vi "tsdb_get_flexray_ecu_properties_by_address_verbose.vi"(8 "error in (no error)":errorcluster caption="错误输入（无错误）", 10 "AAddr":string, 11 "path in":path) -> (0 "error out":errorcluster caption="错误输出", 1 "flexray_ecu_properties_by_address":T1, 2 "function return":i32, 3 "path out":path)   [LabVIEW 2014]
doc: "Function introduction: Obtain Flexray ECU attribute information through address\nCall location\nInput parameter Adder: Address\nADBIndex：\n Database index\nAECUIndex：\n Number of returned signals\nATxFrameCount：\n Returned TX frame rate\nARxFrameCount：\n The number of Rx frames returned\nAName：\n Database Name\nAComment：\n notes\nReturn value 0: Successful execution\nOther values: Failed"
uses:
  Typedef/FlexRay/flexray_ecu_properties_by_address.ctl
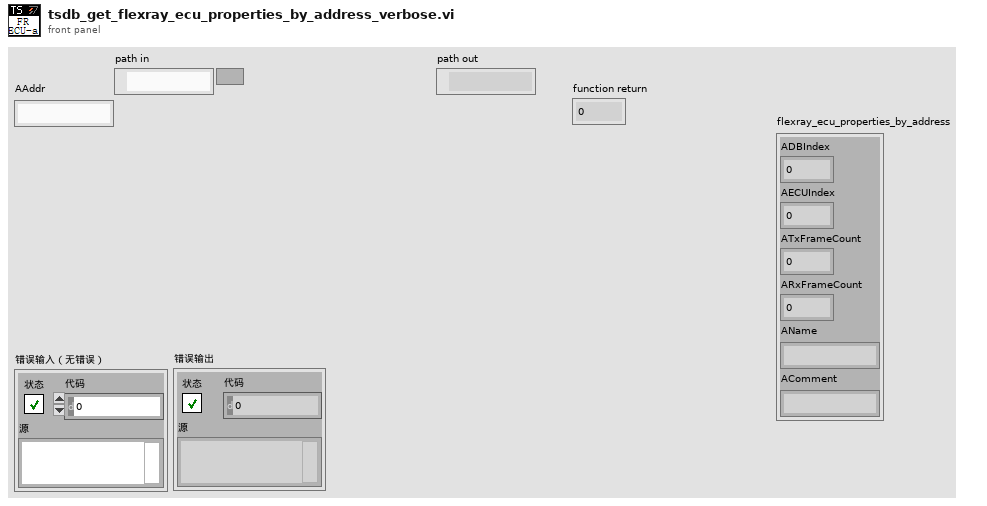
[diagram p1: front panel]
types:
  T1 = typedef "flexray_ecu_properties_by_address.ctl" = cluster{"ADBIndex":i32, "AECUIndex":i32, "ATxFrameCount":i32, "ARxFrameCount":i32, "AName":string, "AComment":string}
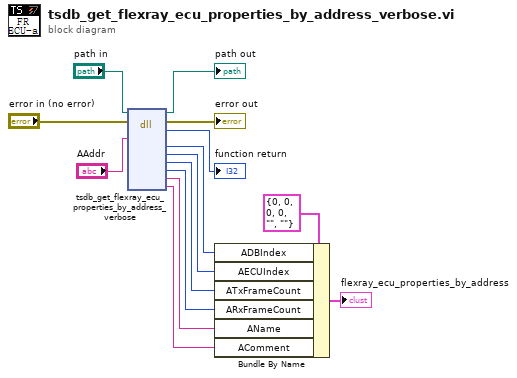
[diagram p0: block diagram]
diagram:
  n1 = dll-call lib="D:/Work/LabVIEW Code/TSMaster Labview SDK/LabVIEW/LabVIEW-TSMasterAPI_CLN/TSMasterAPI_LabVIEW-2024-10-08 14-20-13/Not_organized_vi/TSMaster.*" fn="tsdb_get_flexray_ecu_properties_by_address_verbose"(path in="path in", error in="error in (no error)", "AAddr"="AAddr") -> (path out=→"path out":path, error out=→"error out":errorcluster, "返回类型"=→"function return":i32, "ADBIndex"=w6:i32, "AECUIndex"=w5:i32, "ATxFrameCount"=w4:i32, "ARxFrameCount"=w3:i32, "AName"=w2:string, "AComment"=w1:string)  [unwired: 8 in]
  n2 = Bundle By Name(cluster=T1 {"ADBIndex"=0, "AECUIndex"=0, "ATxFrameCount"=0, "ARxFrameCount"=0, "AName"="", "AComment"=""} ("flexray_ecu_properties_by_address"), "ADBIndex"=w6, "AECUIndex"=w5, "ATxFrameCount"=w4, "ARxFrameCount"=w3, "AName"=w2, "AComment"=w1) -> (→"flexray_ecu_properties_by_address":T1)
